vi "Build Parameters.vi"(10 "Scenarios In":cluster{"Scenario":string, "Parameters":T2}[](array[cluster])) -> (2 "Scenarios out":T1(array[cluster]))   [LabVIEW 2020, in "Param Unit Test.lvclass"]
doc: "This helper function simplifies the syntax of creating parameters."
uses:
  Param Unit Test.lvclass
  Parameters.ctl
  Param Unit Test.lvclass/Param Unit Test.ctl
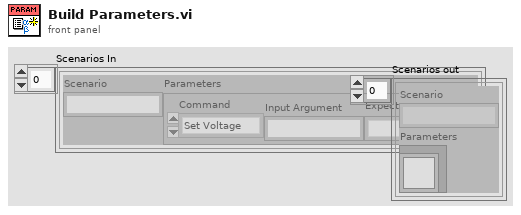
[diagram p1: front panel]
types:
  T1 = cluster{"Scenario":string, "Parameters":refnum<class "Param Unit Test.lvclass">}[]
  T2 = typedef "Param Unit Test.lvclass/Parameters.ctl" = cluster{"Command":enum16{"Set Voltage", "Set Frecuency", "Set Speed", "Set Current"}, "Input Argument":string, "Expected Command":string}
  T3 = cluster{"Scenario":string, "Parameters":refnum<class "Param Unit Test.lvclass">}
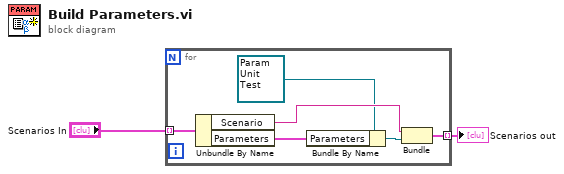
[diagram p0: block diagram]
diagram:
  n1 = for {
    tunnel: [w4] -> w1 mode=indexing
    tunnel: "Scenarios In" -> [w8] mode=indexing
    n2 = Unbundle By Name(w8) -> ("Scenario"=w7:string, "Parameters"=w3:T2)
    n3 = Bundle By Name(cluster=refnum<class "Param Unit Test.lvclass"> refnum ("Parameters"), "Parameters"=w3) -> (w5:refnum<class "Param Unit Test.lvclass">)
    n4 = Bundle("Scenario"=w7, "Parameters"=w5) -> (w4:T3)  [unwired: 1 in]
  }
  "Scenarios out" <- w1
